vi "Change Tag Select DT.vi"(6 "Variant":variant, 8 "error in (no error)":errorcluster, 9 "old values":string[][](array[string]), 10 "object ref in":T2, 11 "Cluster":T3) -> (0 "error out":errorcluster)   [LabVIEW 2013, in "Table Test Editor Node.lvclass"]
uses:
  Table Test Editor Node.lvclass
  Table Manager/Cell Change.ctl
  Table Manager/object ref.ctl
  <vilib>/NI/Tag Bus Data Framework/Configuration Editor/Classes/Engine Parent/Engine Parent Editor Node.lvclass
  <vilib>/NI/Tag Bus Data Framework/Configuration Editor/Classes/Module editor node/module editor node.lvclass
  <vilib>/NI/Tag Bus/tag/Data Type.ctl
  module/configuration/Table Test configuration.lvclass
  module/configuration/Table Test configuration.lvclass/Table Test configuration.ctl
  Table Manager.lvlib
  Table Manager/Table Manager.lvclass
  <vilib>/NI/Tag Bus/tag/tag descriptor.lvclass
panel:
  in  "data type":T1
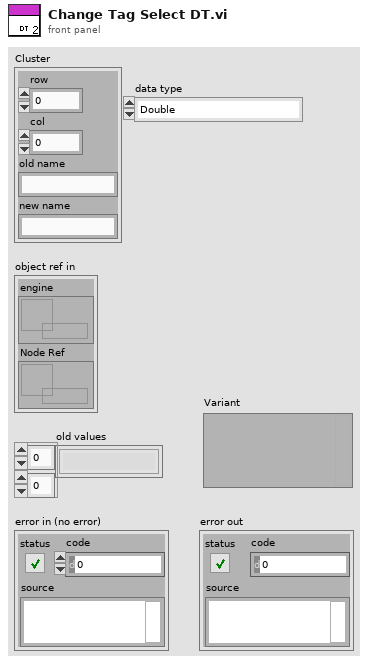
[diagram p1: front panel]
types:
  T1 = typedef "tag bus.lvlib/tag descriptor.lvclass/Data Type.ctl" = enum16{"Double", "Single", "I64", "I32", "I16", "I8", "U64", "U32", "U16", "U8", "Boolean", "String", "Array of Double", "Array of Single", "Array of I64", "Array of I32", "Array of I16", "Array of I8", "Array of U64", "Array of U32", "Array of U16", "Array of U8", "Array of Boolean", "Array of String"}
  T2 = typedef "Table Manager.lvlib/Table Manager.lvclass/object ref.ctl" = cluster{"engine":refnum<data-value>, "Node Ref":refnum<data-value>}
  T3 = typedef "Table Manager.lvlib/Cell Change.ctl" = cluster{"row":i32, "col":i32, "old name":string, "new name":string}
  T4 = typedef "Table Test configuration.lvclass/tag select configuration.ctl" = cluster{"tag select name":string, "data type":T1, "output":refnum<class "TBM channel.lvclass">, "select":refnum<class "TBM channel.lvclass">, "input channels":refnum<class "TBM channel.lvclass">[]}
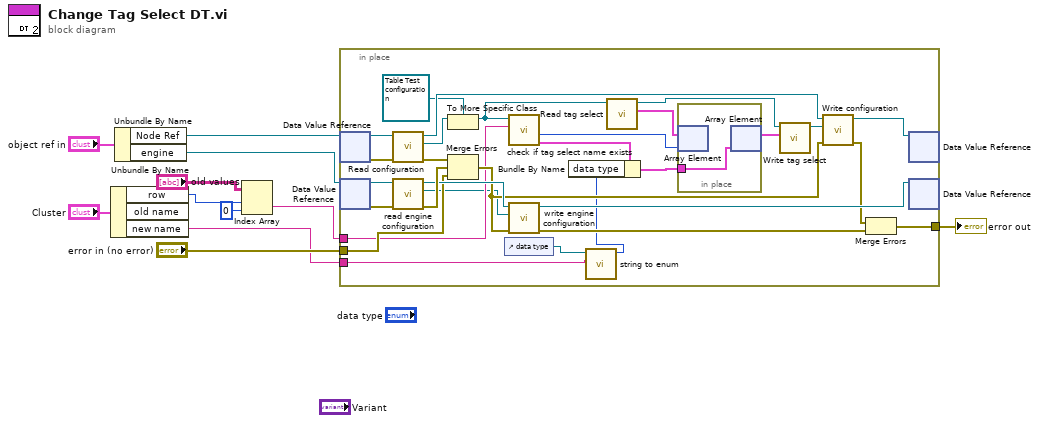
[diagram p0: block diagram]
diagram:
  n1 = Unbundle By Name("Cluster") -> ("row"=w3:i32, "new name"=w5:string)  [unwired: 1 out]
  n2 = Unbundle By Name("object ref in") -> ("Node Ref"=w7:refnum<data-value>, "engine"=w6:refnum<data-value>)
  n3 = Index Array(array="old values", index (row)=w3, index (col)=0 ("disabled index (col)")) -> (element=w1:string)
  n4 = in-place {
    in-place-border: [w33] -> w11
    in-place-border: "error in (no error)" -> [w25]
    in-place-border: w1 -> [w18]
    in-place-border: w5 -> [w14]
    n5 = in-place-dvr #1(w7) -> (w30:refnum<class "module editor node.lvclass">, w32:errorcluster)
    n6 = in-place-dvr #2(w6) -> (w40:refnum<class "Engine Parent Editor Node.lvclass">, w41:errorcluster)
    n7 = call-dynamic "Read configuration.vi"("error in"=w32, "NISE_CEF_serializable node in"=w30) -> ("error out"=w31:errorcluster, "configuration"=w28:refnum<class "NISE_CEF_serializable configuration.lvclass">, "NISE_CEF_serializable node out"=w29:refnum<class "module editor node.lvclass">)  [unwired: 7 in]
    n8 = call <vilib>:"read engine configuration.vi"("error in"=w41, "Engine Parent Editor Node in"=w40) -> ("error out"=w37:errorcluster, "engine configuration"=w15:refnum<class "engine configuration.lvclass">, "Engine Parent Editor Node out"=w36:refnum<class "Engine Parent Editor Node.lvclass">)  [unwired: 7 in]
    n9 = To More Specific Class(target class=refnum<class "Table Test configuration.lvclass"> refnum ("tag select module configuration"), reference=w28) -> (specific class reference=w24:refnum<class "Table Test configuration.lvclass">)  [unwired: 1 in, 1 out]
    n10 = Merge Errors(w31, w37, w25) -> (w27:errorcluster)
    n11 = control-ref of="data type"() -> (w13:refnum<vi>)
    n12 = call "check if tag select name exists.vi"("name to locate"=w18, "tag select module configuration in"=w24) -> ("tag select config"=w19:T4, "index"=w20:i32)  [unwired: 6 in, 2 out]
    n13 = call <vilib>:"write engine configuration.vi"("error in"=w27, "engine configuration"=w15, "Engine Parent Editor Node in"=w36) -> ("error out"=w35:errorcluster, "Engine Parent Editor Node out"=w39:refnum<class "Engine Parent Editor Node.lvclass">)  [unwired: 7 in]
    n14 = call "string to enum.vi"("String"=w14, "Enum"=w13) -> ("Value"=w12:i32)  [unwired: 8 in, 1 out]
    n15 = Bundle By Name(cluster=w19, "data type"=w12) -> (w17:T4)
    n16 = call "Read tag select.vi"("tag select module configuration in"=w24) -> ("tag select"=w23:T4[], "tag select module configuration out"=w21:refnum<class "Table Test configuration.lvclass">)  [unwired: 8 in, 1 out]
    n17 = in-place {
      in-place-border: w17 -> [w42]
      n18 = in-place-array #3(w23, w20) -> ()  [unwired: 1 out]
      n19 = in-place-array #3(w42) -> (w22:T4[])  [unwired: 1 out]
    }
    n20 = call "Write tag select.vi"("tag select"=w22, "tag select module configuration in"=w21) -> ("tag select module configuration out"=w16:refnum<class "Table Test configuration.lvclass">)  [unwired: 8 in, 1 out]
    n21 = call-dynamic "Write configuration.vi"("error in"=w27, "configuration"=w16, "NISE_CEF_serializable node in"=w29) -> ("error out"=w34:errorcluster, "NISE_CEF_serializable node out"=w38:refnum<class "module editor node.lvclass">)  [unwired: 7 in]
    n22 = Merge Errors(w34, w35) -> (w33:errorcluster)
    n23 = in-place-dvr #1(w38) -> ()  [unwired: 2 out]
    n24 = in-place-dvr #2(w39) -> ()  [unwired: 2 out]
  }
  "error out" <- w11
